vi "One Chart Temple.vi"() -> ()   [LabVIEW 2015]
doc: "该连续测量范例项目在队列消息处理器模板的基础上实现。\n\n事件处理循环负责按用户界面操作生成对应的消息。\n\n消息处理循环负责对事件处理循环或其他消息生成的消息进行处理。其中还包括用于采集和记录消息处理循环的子VI，以及用于更新图表的循环。"
uses:
  Settings/Settings.ctl
  Acquisition/Hardware Configuration.ctl
  Logging/Logging Configuration.ctl
  controls/UI Data.ctl
  controls/UI State.ctl
  support/Message Queue/Enqueue Message (Single).vi
  <vilib>/Utility/error.llb/Error Cluster From Error Code.vi
  <vilib>/ErrorRing/Error Ring.xnode
  Acquisition/Acquisition.lvlib
  Logging/Logging.lvlib
  Settings/Settings.lvlib
  support/User Event - Stop/User Event - Stop.lvlib
  support/Message Queue/Message Queue.lvlib
  Motor Control/Motor Control.lvlib
panel:
  out "XY Graph":cluster{"Y":dbl[], "Y":dbl[]}[](graph) caption="XY图"
  in  "清零":bool
  in  "读取":bool
  out "模拟通道5":dbl
  out "模拟通道4":dbl
  out "模拟通道3":dbl
  out "模拟通道2":dbl
  out "模拟通道1":dbl
  out "模拟通道0":dbl
  out "角度":dbl
  in  "计算":bool
  in  "Start":bool caption="开始"
  in  "Stop":bool caption="停止"
  out "Status":string caption="状态"
  in  "Exit":bool caption="退出"
  # "测量项目"
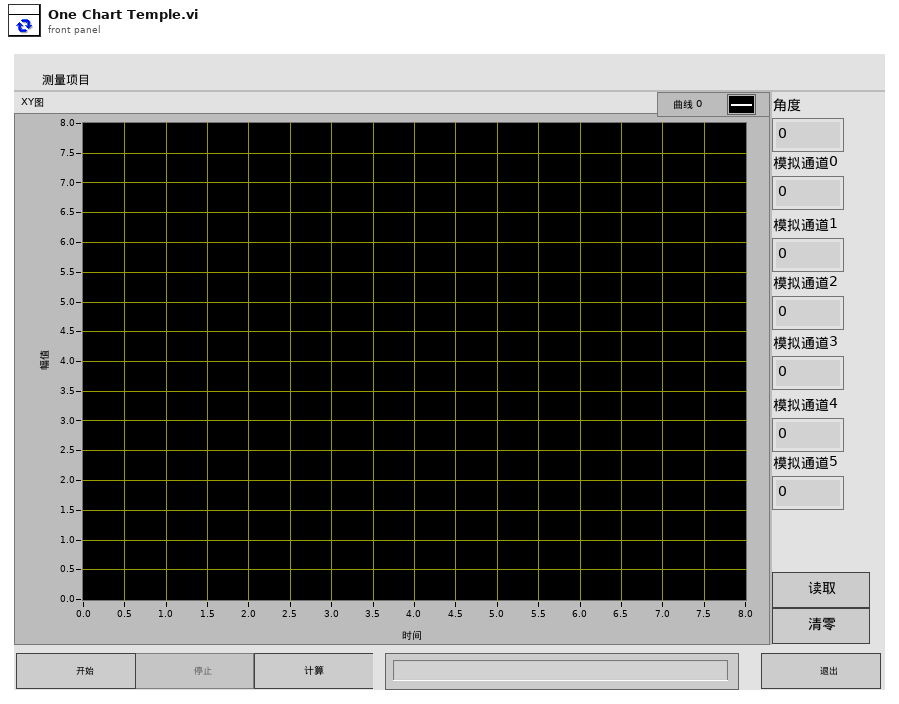
[diagram p1: front panel]
types:
  T1 = typedef "UI State.ctl" = enum16{"Idle", "Acquiring and Logging", "Waiting for Exit", "Waiting for Exit (Acq Stopped)", "Waiting for Exit (Log Stopped)", "Waiting for Stop", "Waiting for Stop (Acq Stopped)", "Waiting for Stop (Log Stopped)"}
  T2 = typedef "UI Data.ctl" = cluster{"Start Ref":refnum<vi>, "Stop Ref":refnum<vi>, "calculate Ref":refnum<vi>, "Status Ref":refnum<vi>, "Exit Ref":refnum<vi>, "Data Ref":refnum<vi>, "read Ref":refnum<vi>, "clean Ref":refnum<vi>}
  T3 = typedef "Settings.lvlib/Settings.ctl" = cluster{"Hardware Configuration":T4, "Logging Configuration":T5}
  T4 = typedef "Acquisition.lvlib/Hardware Configuration.ctl" = cluster{"电压读取设置":cluster{"DAQmx Channel":tag, "Max Input":dbl, "Min Input":dbl, "Sample Rate":dbl, "Sample Number":i32, "DAQmx Task":refnum<k21>}, "角度传感器设置":cluster{"counter":tag, "units":i32, "分辨率":i32, "初始角度":dbl, "DecodingType":i32, "A相端口":tag, "B相端口":tag, "task in":refnum<k21>}}
  T5 = typedef "Logging.lvlib/Logging Configuration.ctl" = cluster{"Log File Base Path":path, "电压传感器转换率":dbl[], "电压传感器本底":dbl[]}
  T6 = typedef "Message Queue.lvlib/All Message Queues.ctl" = cluster{"UI":refnum<queue>, "Acquisition":refnum<queue>, "Logging":refnum<queue>, "MotorCtrl":refnum<queue>, "plot logic":refnum<queue>}
  T7 = enum8{"Enabled", "Disabled", "Disabled and Grayed Out"}
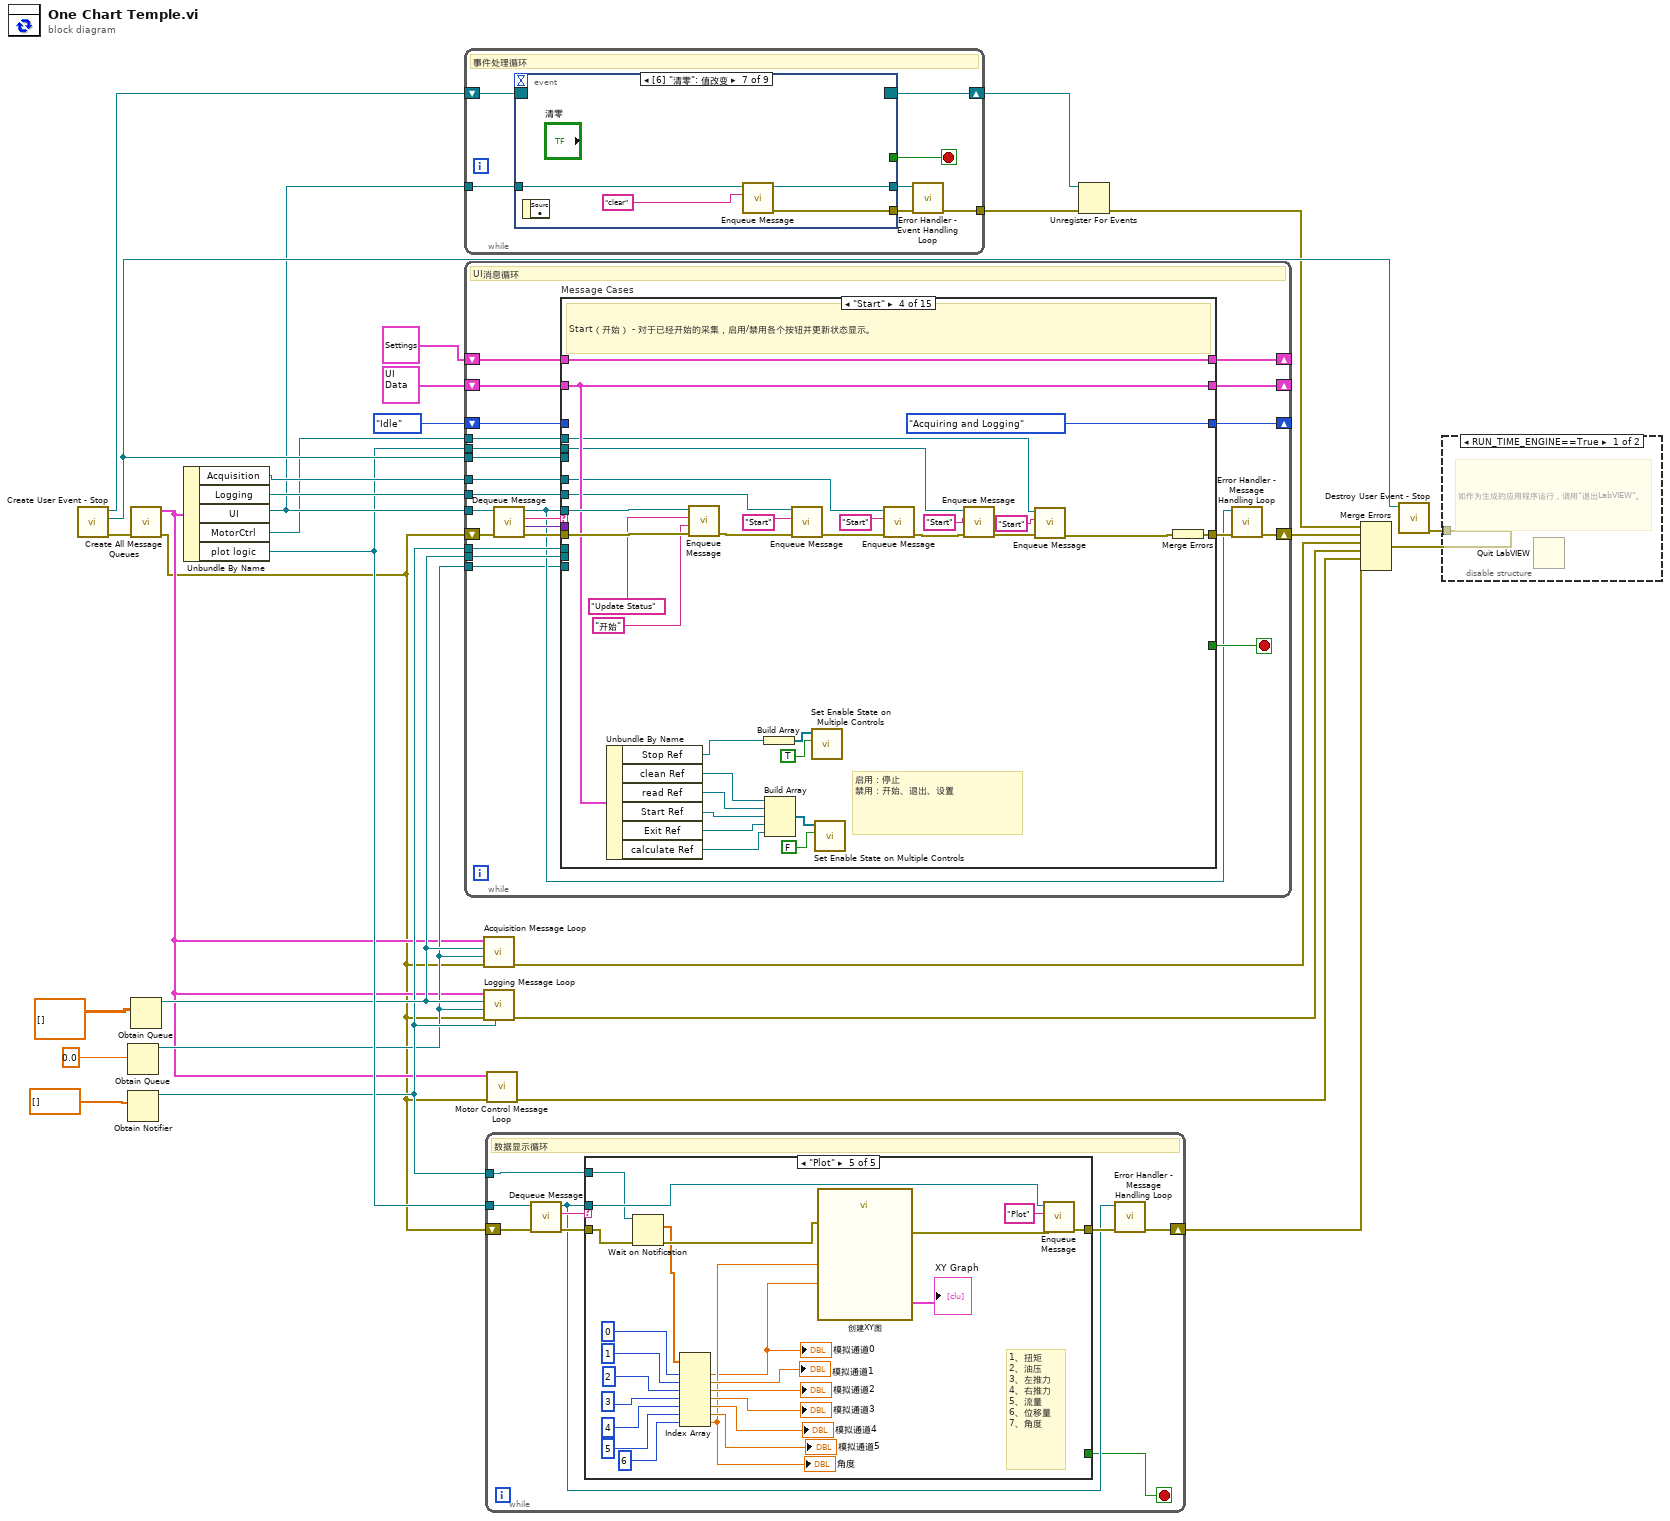
[diagram p0: block diagram]
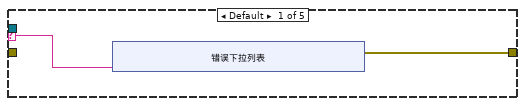
[diagram p3: hidden frame]
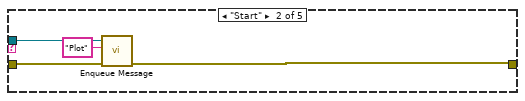
[diagram p4: hidden frame]
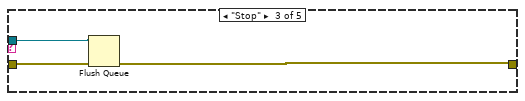
[diagram p5: hidden frame]
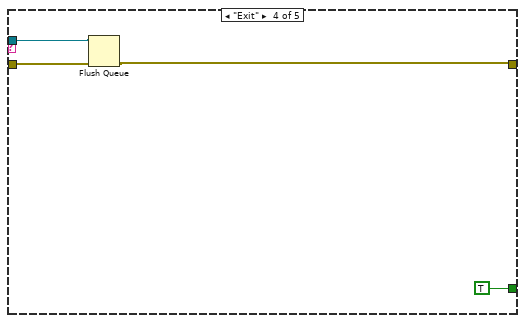
[diagram p6: hidden frame]
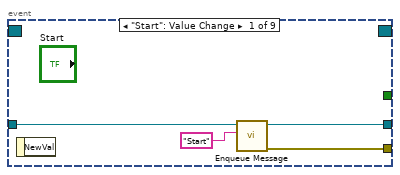
[diagram p7: hidden frame]
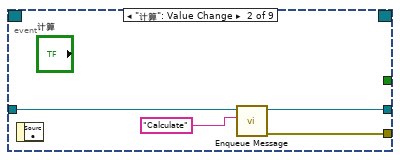
[diagram p8: hidden frame]
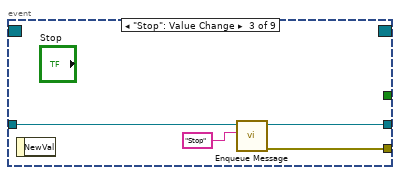
[diagram p9: hidden frame]
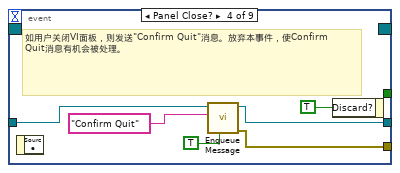
[diagram p10: hidden frame]
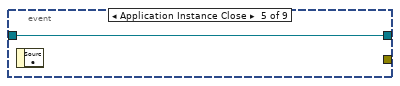
[diagram p11: hidden frame]
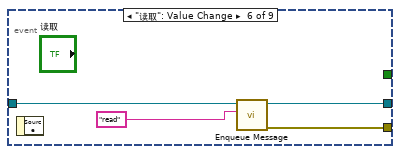
[diagram p12: hidden frame]
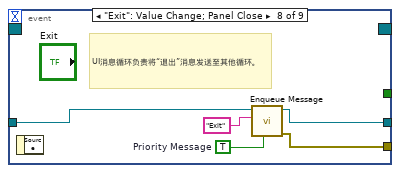
[diagram p13: hidden frame]
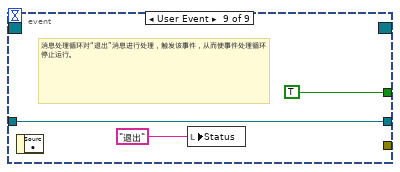
[diagram p14: hidden frame]
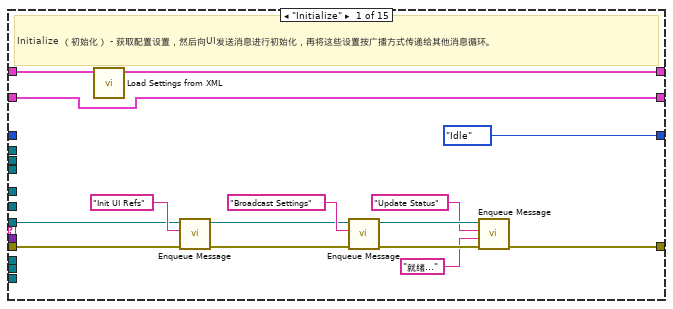
[diagram p15: hidden frame]
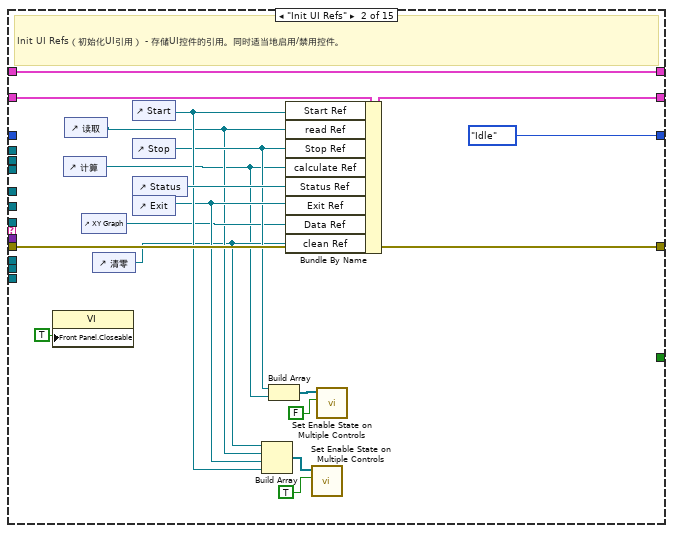
[diagram p16: hidden frame]
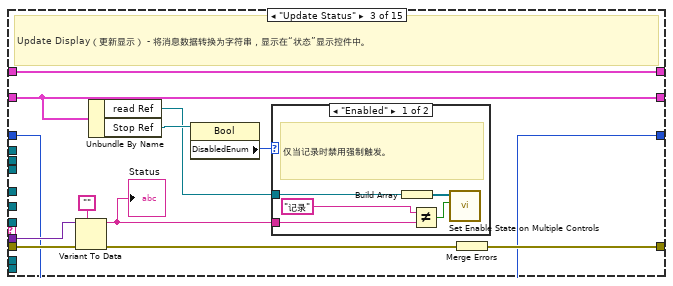
[diagram p17: hidden frame]
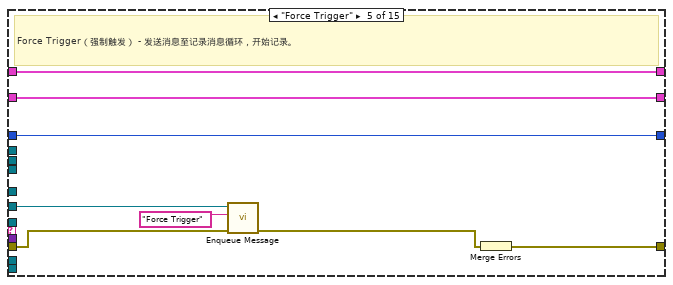
[diagram p19: hidden frame]
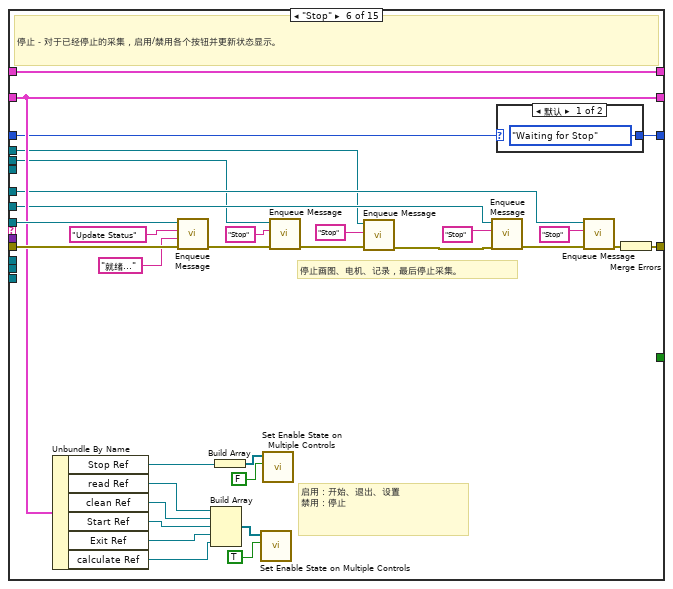
[diagram p20: hidden frame]
diagram:
  n1 = call "Create User Event - Stop.vi"() -> ("error out"=w23:errorcluster, "User Event - Stop"=w25:refnum<user-event>, "Stop Event Registration Refnum"=w26:refnum<event-registration>)  [unwired: 9 in]
  n2 = Obtain Queue(element data type=0.0) -> (queue out=w5:refnum<queue>)  [unwired: 4 in, 2 out]
  n3 = Obtain Notifier(notification data type=dbl[] []) -> (notifier out=w7:refnum<notifier>)  [unwired: 3 in, 2 out]
  n4 = call "Create All Message Queues.vi"("error in (no error)"=w23) -> ("error out"=w3:errorcluster, "Message Queues out"=w4:T6)  [unwired: 9 in]
  n5 = Obtain Queue(element data type=dbl[][] []) -> (queue out=w8:refnum<queue>)  [unwired: 4 in, 2 out]
  n6 = Unbundle By Name(w4) -> ("Acquisition"=w17:refnum<queue>, "Logging"=w16:refnum<queue>, "UI"=w15:refnum<queue>, "MotorCtrl"=w12:refnum<queue>, "plot logic"=w11:refnum<queue>)
  n7 = while {
    tunnel: w15 -> [w35]
    tunnel: [w30] -> w28
    shift-right: [w34] -> w19
    shift-left: w26 -> [w36]
    stop <- w33 stop-if-true
    # "事件处理循环"
    n8 = event shown="[6] \"清零\": 值改变" {
      selector: w36 -> [_ _ _ _ _ _ _ _ _]
      dyn-events: [_ _ _ _ _ _ _ _ _] -> w34
      timeout: _ -> [_ _ _ _ _ _ _ _ _]
      tunnel: [_ _ _ _ _ _ _ _ TRUE ("Discard?")] -> w33
      tunnel: w35 -> [w38 w43 w47 w54 w55 w57 w61 w65 w69]
      tunnel: [w40 w42 w46 w49 _ w59 w63 w68 _] -> w31
      tunnel: [w37 w41 w45 w50 w55 w56 w60 w64 w69] -> w32
      event "Start": Value Change {
        n9 = event-data() -> ()  [unwired: 1 in, 1 out]
        n10 = call-poly "Enqueue Message.vi"("Message"="Start", "Message Queue"=w38) -> ("error out"=w40:errorcluster, "dup Message Queue"=w37:refnum<queue>)  [unwired: 8 in]
      }
      event "计算": Value Change {
        n11 = event-data() -> ()  [unwired: 1 in, 1 out]
        n12 = call-poly "Enqueue Message.vi"("Message"="Calculate", "Message Queue"=w43) -> ("error out"=w42:errorcluster, "dup Message Queue"=w41:refnum<queue>)  [unwired: 8 in]
      }
      event "Stop": Value Change {
        n13 = event-data() -> ()  [unwired: 1 in, 1 out]
        n14 = call-poly "Enqueue Message.vi"("Message"="Stop", "Message Queue"=w47) -> ("error out"=w46:errorcluster, "dup Message Queue"=w45:refnum<queue>)  [unwired: 8 in]
      }
      event Panel Close? {
        # "如用户关闭VI面板，则发送\"Confirm Quit\"消息。放弃本事件，使Confirm Quit消息有机会被处理。"
        n15 = event-data() -> ()  [unwired: 1 in, 1 out]
        n16 = call-poly "Enqueue Message.vi"("Priority Message? (F)"=TRUE, "Message"="Confirm Quit", "Message Queue"=w54) -> ("error out"=w49:errorcluster, "dup Message Queue"=w50:refnum<queue>)  [unwired: 7 in]
        n17 = event-data("Discard?"=TRUE) -> ()  [unwired: 1 in, 1 out]
      }
      event Application Instance Close {
        n18 = event-data() -> ()  [unwired: 1 in, 1 out]
      }
      event "读取": Value Change {
        n19 = event-data() -> ()  [unwired: 1 in, 1 out]
        n20 = call-poly "Enqueue Message.vi"("Message"="read", "Message Queue"=w57) -> ("error out"=w59:errorcluster, "dup Message Queue"=w56:refnum<queue>)  [unwired: 8 in]
      }
      event "清零": Value Change {
        n21 = event-data() -> ()  [unwired: 1 in, 1 out]
        n22 = call-poly "Enqueue Message.vi"("Message"="clear", "Message Queue"=w61) -> ("error out"=w63:errorcluster, "dup Message Queue"=w60:refnum<queue>)  [unwired: 8 in]
      }
      event "Exit": Value Change; Panel Close {
        w66 = TRUE  # Priority Message
        # "UI消息循环负责将“退出”消息发送至其他循环。"
        n23 = event-data() -> ()  [unwired: 1 in, 1 out]
        n24 = call-poly "Enqueue Message.vi"("Priority Message? (F)"=w66, "Message"="Exit", "Message Queue"=w65) -> ("error out"=w68:errorcluster, "dup Message Queue"=w64:refnum<queue>)  [unwired: 7 in]
      }
      event User Event {
        # "消息处理循环对“退出”消息进行处理，触发该事件，从而使事件处理循环停止运行。"
        n25 = event-data() -> ()  [unwired: 1 in, 1 out]
        n26 = local write "Status"("退出" ("Exit String")) -> ()
      }
    }
    n27 = call "Error Handler - Event Handling Loop.vi"("error in (no error)"=w31, "Message Queue"=w32) -> ("dup error in"=w30:errorcluster)  [unwired: 8 in, 1 out]
  }
  n28 = while {
    tunnel: w15 -> [w88]
    tunnel: w25 -> [w93]
    shift-right: [w78] -> w29
    shift-left: w3 -> [w92]
    shift-right: [w87] -> _
    shift-left: T3 {"Hardware Configuration"={"电压读取设置"={"DAQmx Channel"="", "Max Input"=0.0, "Min Input"=0.0, "Sample Rate"=0.0, "Sample Number"=0, "DAQmx Task"=""}, "角度传感器设置"={"counter"="Dev1/ctr0", "units"=10146, "分辨率"=0, "初始角度"=0.0, "DecodingType"=10092, "A相端口"="/Dev1/PFI8", "B相端口"="/Dev1/PFI8", "task in"=""}}, "Logging Configuration"={"Log File Base Path"=path "", "电压传感器转换率"=[], "电压传感器本底"=[]}} ("Settings") -> [w86]
    shift-right: [w84] -> _
    shift-left: T2 {"Start Ref"=refnum, "Stop Ref"=refnum, "calculate Ref"=refnum, "Status Ref"=refnum, "Exit Ref"=refnum, "Data Ref"=refnum, "read Ref"=refnum, "clean Ref"=refnum} ("Measurement UI Controls") -> [w85]
    tunnel: w17 -> [w83]
    tunnel: w16 -> [w82]
    tunnel: w7 -> [w81]
    tunnel: w8 -> [w80]
    shift-right: [w75] -> _
    shift-left: UI_State."Idle" ("UI State") -> [w76]
    tunnel: w12 -> [w72]
    tunnel: w11 -> [w73]
    tunnel: w5 -> [w74]
    stop <- w94 stop-if-true
    # "UI消息循环"
    n29 = call "Dequeue Message.vi"("error in (no error)"=w92, "Message Queue"=w88) -> ("error out"=w91:errorcluster, "Message Data"=w89:variant, "Message"=w90:string, "dup Message Queue"=w77:refnum<queue>)  [unwired: 6 in]
    n30 = case "Message Cases" shown="\"Start\"" w90 {
      selector: w90 -> [_ _ _ _ _ _ _ _ _ _ _ _ _ _ w362]
      tunnel: w77 -> [w99 _ _ w174 _ w214 w218 w243 _ w285 w300 w310 w345 _ _]
      tunnel: w91 -> [w98 w127 w138 w173 w180 w213 w220 w245 w273 w287 w304 w309 w353 w360 _]
      tunnel: [w105 w127 w139 w175 w183 w215 w219 w244 w279 w282 w295 w308 w354 w359 w363] -> w79
      tunnel: [_ _ _ _ _ _ _ _ _ _ _ _ TRUE _ _] -> w94
      tunnel: w89 -> [_ _ w137 _ _ _ _ _ _ _ w303 _ _ _ _]
      tunnel: w93 -> [_ _ _ _ _ _ _ _ _ _ _ _ w352 _ _]
      tunnel: [w108 w126 w134 w172 w182 w212 w224 w249 w277 w284 w306 w313 w350 w358 w365] -> w87
      tunnel: w86 -> [w109 w126 w134 w172 w182 w212 w224 w249 w277 w288 w306 w313 w350 w358 w365]
      tunnel: w85 -> [w101 w125 w133 w169 w181 w209 w223 w248 w271 w281 w305 w312 w348 w357 w364]
      tunnel: [w101 w124 w133 w169 w181 w209 w223 w248 w271 w281 w305 w312 w348 w357 w364] -> w84
      tunnel: w83 -> [_ _ _ w157 _ w197 _ _ w270 _ _ _ w347 _ _]
      tunnel: w82 -> [_ _ _ w159 w177 w200 _ _ w269 _ _ _ w346 _ _]
      tunnel: w81 -> [_ _ _ _ _ _ _ _ _ _ _ _ w344 _ _]
      tunnel: w80 -> [_ _ _ _ _ _ _ _ _ _ _ _ w341 _ _]
      tunnel: w76 -> [_ _ w128 _ w176 w195 w222 w247 w268 w280 w294 w311 _ w356 w361]
      tunnel: [UI_State."Idle" ("UI State") UI_State."Idle" ("UI State") w128 UI_State."Acquiring and Logging" ("UI State") w176 w194 w221 w246 w268 w280 w294 w307 UI_State."Idle" ("UI State") w356 w361] -> w75
      tunnel: w74 -> [_ _ _ _ _ _ _ _ _ _ _ _ w335 _ _]
      tunnel: w73 -> [_ _ _ w151 _ w187 _ _ _ _ _ _ _ _ _]
      tunnel: w72 -> [_ _ _ w147 _ w185 _ _ _ _ _ _ _ _ _]
      frame "Initialize" {
        # "Initialize （初始化） - 获取配置设置，然后向UI发送消息进行初始化，再将这些设置按广播方式传递给其他消息循环。"
        n31 = call "Load Settings from XML.vi"("Settings in"=w109) -> ("Settings out"=w108:T3)  [unwired: 9 in, 1 out]
        n32 = call-poly "Enqueue Message.vi"("error in (no error)"=w98, "Message"="Init UI Refs", "Message Queue"=w99) -> ("error out"=w96:errorcluster, "dup Message Queue"=w97:refnum<queue>)  [unwired: 7 in]
        n33 = call-poly "Enqueue Message.vi"("error in (no error)"=w96, "Message"="Broadcast Settings", "Message Queue"=w97) -> ("error out"=w107:errorcluster, "dup Message Queue"=w106:refnum<queue>)  [unwired: 7 in]
        n34 = call-poly "Enqueue Message.vi"("error in (no error)"=w107, "Message Data"="就绪..." ("Ready..."), "Message"="Update Status", "Message Queue"=w106) -> ("error out"=w105:errorcluster)  [unwired: 6 in, 1 out]
      }
      frame "Init UI Refs" {
        # "Init UI Refs（初始化UI引用） - 存储UI控件的引用。同时适当地启用/禁用控件。"
        n35 = property class="VI"("Front Panel.Closeable"=TRUE ("Front Panel Window:Closeable")) -> ()  [unwired: 2 in, 2 out]
        n36 = control-ref of="计算"() -> (w110:refnum<vi>)
        n37 = control-ref of="读取"() -> (w112:refnum<vi>)
        n38 = control-ref of="XY Graph"() -> (w113:refnum<vi>)
        n39 = control-ref of="清零"() -> (w111:refnum<vi>)
        n40 = control-ref of="Start"() -> (w120:refnum<vi>)
        n41 = control-ref of="Stop"() -> (w116:refnum<vi>)
        n42 = control-ref of="Status"() -> (w121:refnum<vi>)
        n43 = control-ref of="Exit"() -> (w117:refnum<vi>)
        n44 = Build Array(w111, w112, w117, w120) -> (w119:refnum<vi>[])
        n45 = Build Array(w116, w110) -> (w115:refnum<vi>[])
        n46 = Bundle By Name(cluster=w125, "Start Ref"=w120, "read Ref"=w112, "Stop Ref"=w116, "calculate Ref"=w110, "Status Ref"=w121, "Exit Ref"=w117, "Data Ref"=w113, "clean Ref"=w111) -> (w124:T2)
        n47 = call "Set Enable State on Multiple Controls.vi"("Enable?"=TRUE, "Controls"=w119) -> ()  [unwired: 10 in]
        n48 = call "Set Enable State on Multiple Controls.vi"("Enable?"=FALSE, "Controls"=w115) -> ()  [unwired: 10 in]
      }
      frame "Update Status" {
        # "Update Display（更新显示） - 将消息数据转换为字符串，显示在“状态”显示控件中。"
        n49 = Variant To Data(error in=w138, type="", Variant=w137) -> (data=w130:string, error out=w135:errorcluster)
        "Status" <- w130
        n50 = Unbundle By Name(w133) -> ("read Ref"=w129:refnum<vi>, "Stop Ref"=w132:refnum<vi>)
        n51 = property class="Bool"(reference=w132) -> ("DisabledEnum"=w131:T7)  [unwired: 1 in, 2 out]
        n52 = case shown="\"Enabled\"" w131 {
          tunnel: w130 -> [w142 _]
          tunnel: w129 -> [w143 _]
          frame "Enabled" {
            # "仅当记录时禁用强制触发。"
            n53 = Build Array(w143) -> (w144:refnum<vi>[])
            n54 = Not Equal?(x="记录" ("Logging"), y=w142) -> (x != y?=w140:bool)
            n55 = call "Set Enable State on Multiple Controls.vi"("Enable?"=w140, "Controls"=w144) -> ()  [unwired: 10 in]
          }
          frame "Disabled", Default {
          }
        }
        n56 = Merge Errors(w135) -> (w139:errorcluster)
      }
      frame "Start" {
        # "启用：停止\n禁用：开始、退出、设置"
        # "Start（开始） - 对于已经开始的采集，启用/禁用各个按钮并更新状态显示。"
        n57 = Unbundle By Name(w169) -> ("Stop Ref"=w152:refnum<vi>, "clean Ref"=w153:refnum<vi>, "read Ref"=w154:refnum<vi>, "Start Ref"=w164:refnum<vi>, "Exit Ref"=w163:refnum<vi>, "calculate Ref"=w162:refnum<vi>)
        n58 = call-poly "Enqueue Message.vi"("error in (no error)"=w173, "Message Data"="开始" ("Waiting for trigger"), "Message"="Update Status", "Message Queue"=w174) -> ("error out"=w161:errorcluster)  [unwired: 6 in, 1 out]
        n59 = Build Array(w152) -> (w166:refnum<vi>[])
        n60 = Build Array(w153, w154, w164, w163, w162) -> (w167:refnum<vi>[])
        n61 = call-poly "Enqueue Message.vi"("error in (no error)"=w161, "Message"="Start", "Message Queue"=w159) -> ("error out"=w158:errorcluster)  [unwired: 7 in, 1 out]
        n62 = call "Set Enable State on Multiple Controls.vi"("Enable?"=TRUE, "Controls"=w166) -> ()  [unwired: 10 in]
        n63 = call "Set Enable State on Multiple Controls.vi"("Enable?"=FALSE, "Controls"=w167) -> ()  [unwired: 10 in]
        n64 = call-poly "Enqueue Message.vi"("error in (no error)"=w158, "Message"="Start", "Message Queue"=w157) -> ("error out"=w149:errorcluster)  [unwired: 7 in, 1 out]
        n65 = call-poly "Enqueue Message.vi"("error in (no error)"=w149, "Message"="Start", "Message Queue"=w151) -> ("error out"=w148:errorcluster)  [unwired: 7 in, 1 out]
        n66 = call-poly "Enqueue Message.vi"("error in (no error)"=w148, "Message"="Start", "Message Queue"=w147) -> ("error out"=w145:errorcluster)  [unwired: 7 in, 1 out]
        n67 = Merge Errors(w145) -> (w175:errorcluster)
      }
      frame "Force Trigger" {
        # "Force Trigger（强制触发） - 发送消息至记录消息循环，开始记录。"
        n68 = call-poly "Enqueue Message.vi"("error in (no error)"=w180, "Message"="Force Trigger", "Message Queue"=w177) -> ("error out"=w179:errorcluster)  [unwired: 7 in, 1 out]
        n69 = Merge Errors(w179) -> (w183:errorcluster)
      }
      frame "Stop" {
        # "停止画图、电机、记录，最后停止采集。"
        # "启用：开始、退出、设置\n禁用：停止"
        # "停止－对于已经停止的采集，启用/禁用各个按钮并更新状态显示。"
        n70 = Unbundle By Name(w209) -> ("Stop Ref"=w191:refnum<vi>, "read Ref"=w192:refnum<vi>, "clean Ref"=w193:refnum<vi>, "Start Ref"=w204:refnum<vi>, "Exit Ref"=w203:refnum<vi>, "calculate Ref"=w202:refnum<vi>)
        n71 = call-poly "Enqueue Message.vi"("error in (no error)"=w213, "Message Data"="就绪..." ("Ready..."), "Message"="Update Status", "Message Queue"=w214) -> ("error out"=w190:errorcluster)  [unwired: 6 in, 1 out]
        n72 = Build Array(w192, w193, w204, w203, w202) -> (w207:refnum<vi>[])
        n73 = Build Array(w191) -> (w206:refnum<vi>[])
        n74 = call "Set Enable State on Multiple Controls.vi"("Enable?"=TRUE, "Controls"=w207) -> ()  [unwired: 10 in]
        n75 = call "Set Enable State on Multiple Controls.vi"("Enable?"=FALSE, "Controls"=w206) -> ()  [unwired: 10 in]
        n76 = call-poly "Enqueue Message.vi"("error in (no error)"=w190, "Message"="Stop", "Message Queue"=w187) -> ("error out"=w189:errorcluster)  [unwired: 7 in, 1 out]
        n77 = call-poly "Enqueue Message.vi"("error in (no error)"=w189, "Message"="Stop", "Message Queue"=w185) -> ("error out"=w188:errorcluster)  [unwired: 7 in, 1 out]
        n78 = call-poly "Enqueue Message.vi"("error in (no error)"=w188, "Message"="Stop", "Message Queue"=w200) -> ("error out"=w199:errorcluster)  [unwired: 7 in, 1 out]
        n79 = case shown="默认" w195 {
          selector: w195 -> [_ w217]
          tunnel: [UI_State."Waiting for Stop" ("UI State") w217] -> w194
          frame Default {
          }
          frame "Waiting for Exit" {
          }
        }
        n80 = call-poly "Enqueue Message.vi"("error in (no error)"=w199, "Message"="Stop", "Message Queue"=w197) -> ("error out"=w198:errorcluster)  [unwired: 7 in, 1 out]
        n81 = Merge Errors(w198) -> (w215:errorcluster)
      }
      frame "Acquisition Stopped" {
        # "此处代码用于确定采集停止时采取何种操作。"
        n82 = case shown="\"Waiting for Stop (Log Stopped)\"" w222 {
          selector: w222 -> [w226 _ _ _ _]
          tunnel: [w226 UI_State."Waiting for Exit (Acq Stopped)" ("UI State") UI_State."Waiting for Stop (Acq Stopped)" ("UI State") UI_State."Idle" ("UI State") UI_State."Idle" ("UI State")] -> w221
          tunnel: w220 -> [w225 w227 w229 w235 w241]
          tunnel: [w225 w227 w229 w234 w240] -> w219
          tunnel: w218 -> [_ _ _ w233 w239]
          frame Default {
          }
          frame "Waiting for Exit", "Waiting for Exit (Acq Stopped)" {
          }
          frame "Waiting for Stop", "Waiting for Stop (Acq Stopped)" {
          }
          frame "Waiting for Exit (Log Stopped)" {
            # "如果正在等待退出且记录已结束，“采集停止”消息表示应退出。"
            n83 = call-poly "Enqueue Message.vi"("Priority Message? (F)"=TRUE, "error in (no error)"=w235, "Message"="Exit", "Message Queue"=w233) -> ("error out"=w234:errorcluster)  [unwired: 6 in, 1 out]
          }
          frame "Waiting for Stop (Log Stopped)" {
            # "当前状态为等待停止时，如已停止记录，则收到\"Acquisition Stopped\"消息时即可停止。"
            n84 = call-poly "Enqueue Message.vi"("error in (no error)"=w241, "Message Data"="Ready..." ("Message"), "Message"="Update Status", "Message Queue"=w239) -> ("error out"=w240:errorcluster)  [unwired: 6 in, 1 out]
          }
        }
      }
      frame "Logging Stopped" {
        # "此处代码用于确定记录停止时采取何种操作。"
        n85 = case shown="\"Waiting for Stop (Acq Stopped)\"" w247 {
          selector: w247 -> [w251 _ _ _ _]
          tunnel: [w251 UI_State."Waiting for Exit (Log Stopped)" ("UI State") UI_State."Waiting for Stop (Log Stopped)" ("UI State") UI_State."Idle" ("UI State") UI_State."Idle" ("UI State")] -> w246
          tunnel: w245 -> [w250 w252 w254 w260 w266]
          tunnel: [w250 w252 w254 w259 w265] -> w244
          tunnel: w243 -> [_ _ _ w258 w264]
          frame Default {
          }
          frame "Waiting for Exit", "Waiting for Exit (Log Stopped)" {
          }
          frame "Waiting for Stop", "Waiting for Stop (Log Stopped)" {
          }
          frame "Waiting for Exit (Acq Stopped)" {
            # "如果正在等待退出且采集已结束，“记录停止”消息表示应退出。"
            n86 = call-poly "Enqueue Message.vi"("Priority Message? (F)"=TRUE, "error in (no error)"=w260, "Message"="Exit", "Message Queue"=w258) -> ("error out"=w259:errorcluster)  [unwired: 6 in, 1 out]
          }
          frame "Waiting for Stop (Acq Stopped)" {
            # "如果正在等待停止且采集已结束，“记录停止”消息表示应停止。"
            n87 = call-poly "Enqueue Message.vi"("error in (no error)"=w266, "Message Data"="Ready..." ("Message"), "Message"="Update Status", "Message Queue"=w264) -> ("error out"=w265:errorcluster)  [unwired: 6 in, 1 out]
          }
        }
      }
      frame "Broadcast settings" {
        w272 = "Update Settings" ("Message")
        # "向“记录和采集”消息队列发送“更新设置”消息。"
        n88 = Unbundle By Name(w277) -> ("Hardware Configuration"=w276:T4, "Logging Configuration"=w275:T5)
        n89 = call-poly "Enqueue Message.vi"("Message Data"=w276, "Message"=w272, "Message Queue"=w270) -> ("error out"=w278:errorcluster)  [unwired: 7 in, 1 out]
        n90 = call-poly "Enqueue Message.vi"("error in (no error)"=w278, "Message Data"=w275, "Message"=w272, "Message Queue"=w269) -> ("error out"=w274:errorcluster)  [unwired: 6 in, 1 out]
        n91 = Merge Errors(w274, w273) -> (w279:errorcluster)
      }
      frame "Launch Settings Dialog" {
        # "用户单击“设置”按钮时，启动设置对话框。"
        n92 = call "Settings Dialog.vi"("error in (no error)"=w287, "Settings in"=w288) -> ("error out"=w283:errorcluster, "Cancelled?"=w286:bool, "Settings out"=w284:T3)  [unwired: 6 in, 1 out]
        n93 = case shown="假" w286 {
          tunnel: w285 -> [w292 _]
          tunnel: w283 -> [w291 w293]
          tunnel: [w290 w293] -> w282
          frame False {
            n94 = call-poly "Enqueue Message.vi"("error in (no error)"=w291, "Message"="Broadcast Settings", "Message Queue"=w292) -> ("error out"=w290:errorcluster)  [unwired: 7 in, 1 out]
          }
          frame True {
          }
        }
      }
      frame "Error" {
        # "Error - 检查错误消息数据及其响应。该消息由应用程序各循环结束处的“错误处理”VI发送。"
        n95 = Variant To Data(error in=w304, type=errorcluster {"status"=FALSE, "code"=0, "source"=""} ("error out"), Variant=w303) -> (data=w301:errorcluster, error out=w297:errorcluster)
        n96 = call <vilib>:"Simple Error Handler.vi"("error in (no error)"=w301) -> ()  [unwired: 4 in, 5 out]
        n97 = call-poly "Enqueue Message.vi"("Priority Message? (F)"=TRUE, "Message"="Exit", "Message Queue"=w300) -> ("error out"=w296:errorcluster)  [unwired: 7 in, 1 out]
        n98 = Merge Errors(w296, w297) -> (w295:errorcluster)
      }
      frame "Confirm Quit" {
        # "Confirm Quit - 该消息用于确认用户是否需要退出应用程序。"
        n99 = case shown="\"Acquiring and Logging\"" w311 {
          tunnel: w310 -> [w318 w324]
          tunnel: w309 -> [w317 w322]
          tunnel: [w314 w321] -> w308
          tunnel: [UI_State."Idle" ("UI State") w320] -> w307
          frame Default {
            # "如收到'Confirm Quit'消息时系统处于空闲状态，则不需要弹出确认提示。"
            n100 = call-poly "Enqueue Message.vi"("Priority Message? (F)"=TRUE, "error in (no error)"=w317, "Message"="Exit", "Message Queue"=w318) -> ("error out"=w314:errorcluster)  [unwired: 6 in, 1 out]
          }
          frame "Acquiring and Logging" {
            n101 = Two Button Dialog(message="采集仍在执行中，是否确定退出？" ("Confirm Quit Message"), 1:"否" ("No"), 2:"是" ("Yes")) -> (T button?=w323:bool)
            n102 = case shown="真" w323 {
              tunnel: w324 -> [_ w334]
              tunnel: w322 -> [w328 w333]
              tunnel: [w328 w332] -> w321
              tunnel: [UI_State."Acquiring and Logging" ("UI State") UI_State."Waiting for Exit" ("UI State")] -> w320
              frame False {
                # "用户不希望退出。"
              }
              frame True {
                n103 = call-poly "Enqueue Message.vi"("error in (no error)"=w333, "Message"="Stop", "Message Queue"=w334) -> ("error out"=w332:errorcluster)  [unwired: 7 in, 1 out]
              }
            }
          }
        }
      }
      frame "Exit" {
        w349 = "Exit" ("Message")
        # "不必检查错误输出。采集和记录队列可能已被释放。"
        # "停止VI。"
        # "Exit（退出）－触发用户事件，使“事件处理”循环停止运行。同时向“采集和记录”循环发送“退出”消息。"
        n104 = Release Queue(queue=w345, error in (no error)=w353) -> (error out=w343:errorcluster)  [unwired: 1 in, 2 out]
        n105 = call "Fire User Event - Stop.vi"("User Event - Stop"=w352) -> ("error out"=w351:errorcluster)  [unwired: 10 in]
        n106 = Release Notifier(notifier=w344, error in (no error)=w343) -> (error out=w342:errorcluster)  [unwired: 1 in, 2 out]
        n107 = Release Queue(queue=w341, error in (no error)=w342) -> (error out=w337:errorcluster)  [unwired: 1 in, 2 out]
        n108 = call-poly "Enqueue Message.vi"("Priority Message? (F)"=TRUE, "Message"=w349, "Message Queue"=w347) -> ()  [unwired: 7 in, 2 out]
        n109 = Release Queue(queue=w335, error in (no error)=w337) -> (error out=w336:errorcluster)  [unwired: 1 in, 2 out]
        n110 = call-poly "Enqueue Message.vi"("Priority Message? (F)"=TRUE, "Message"=w349, "Message Queue"=w346) -> ()  [unwired: 7 in, 2 out]
        n111 = Merge Errors(w351, w336) -> (w354:errorcluster)
      }
      frame "---Copy This Frame---" {
        # "如需创建新消息，可创建该帧的副本。在副本中，将本注释更改为对应消息的注释。"
        n112 = Merge Errors(w360) -> (w359:errorcluster)
      }
      frame Default {
        # "如得到的消息未经任何分支定义，则运行“默认”分支。输出程序错误。"
        n113 = xnode "错误下拉列表"("参数 0"=w362) -> ("错误输出"=w363:errorcluster)
      }
    }
    n114 = call "Error Handler - Message Handling Loop.vi"("error in (no error)"=w79, "Message Queue"=w77) -> ("dup error in"=w78:errorcluster)  [unwired: 8 in, 1 out]
  }
  n115 = call "Acquisition Message Loop.vi"("error in (no error)"=w3, "Angle Data Queue"=w5, "Analog Data Queue"=w8, "Message Queues"=w4) -> ("error out"=w24:errorcluster)  [unwired: 7 in]
  n116 = call "Logging Message Loop.vi"("数据通知器"=w7, "error in (no error)"=w3, "Angle Data Queue"=w5, "Analog Data Queue"=w8, "Message Queues"=w4) -> ("error out"=w22:errorcluster)  [unwired: 6 in]
  n117 = while "Data Display Loop" {
    tunnel: w7 -> [w374]
    tunnel: w11 -> [w381]
    shift-right: [w376] -> w1
    shift-left: w3 -> [w380]
    stop <- w373 stop-if-true
    # "数据显示循环"
    n118 = call "Dequeue Message.vi"("error in (no error)"=w380, "Message Queue"=w381) -> ("error out"=w378:errorcluster, "Message"=w377:string, "dup Message Queue"=w375:refnum<queue>)  [unwired: 6 in, 1 out]
    n119 = case shown="\"Plot\"" w377 {
      selector: w377 -> [w382 _ _ _ _]
      tunnel: [w383 w391 w396 w399 w405] -> w379
      tunnel: w378 -> [_ w394 w397 w401 w421]
      tunnel: w375 -> [_ w393 w395 w400 w424]
      tunnel: w374 -> [_ _ _ _ w422]
      tunnel: [_ _ _ TRUE _] -> w373
      frame Default {
        n120 = xnode "错误下拉列表"("参数 0"=w382) -> ("错误输出"=w383:errorcluster)
      }
      frame "Start" {
        n121 = call-poly "Enqueue Message.vi"("error in (no error)"=w394, "Message"="Plot", "Message Queue"=w393) -> ("error out"=w391:errorcluster)  [unwired: 7 in, 1 out]
      }
      frame "Stop" {
        n122 = Flush Queue(queue=w395, error in (no error)=w397) -> (error out=w396:errorcluster)  [unwired: 2 out]
      }
      frame "Exit" {
        n123 = Flush Queue(queue=w400, error in (no error)=w401) -> (error out=w399:errorcluster)  [unwired: 2 out]
      }
      frame "Plot" {
        # "1、扭矩\n2、油压\n3、左推力\n4、右推力\n5、流量\n6、位移量\n7、角度"
        n124 = Wait on Notification(notifier=w422, error in (no error)=w421) -> (notification=w402:dbl[], error out=w407:errorcluster)  [unwired: 2 in, 2 out]
        n125 = Index Array(array=w402, index #1=0 ("索引"), index #2=1 ("索引"), index #3=2 ("索引"), index #4=3 ("索引"), index #5=4 ("索引"), index #6=5 ("索引"), index #7=6 ("索引")) -> (element #1=w403:dbl, element #2=→"模拟通道1":dbl, element #3=→"模拟通道2":dbl, element #4=→"模拟通道3":dbl, element #5=→"模拟通道4":dbl, element #6=→"模拟通道5":dbl, element #7=w404:dbl)
        "角度" <- w404
        "模拟通道0" <- w403
        n126 = call "创建XY图"("error in (no error)"=w407, "Y Input"=w403, "X Input"=w404) -> ("error out"=w406:errorcluster, "XY Graph"=→"XY Graph":cluster{"X":dbl[], "Y":dbl[]}[])  [unwired: 7 in]
        n127 = call-poly "Enqueue Message.vi"("error in (no error)"=w406, "Message"="Plot", "Message Queue"=w424) -> ("error out"=w405:errorcluster)  [unwired: 7 in, 1 out]
      }
    }
    n128 = call "Error Handler - Message Handling Loop.vi"("error in (no error)"=w379, "Message Queue"=w375) -> ("dup error in"=w376:errorcluster)  [unwired: 8 in, 1 out]
  }
  n129 = call "Motor Control Message Loop.vi"("error in (no error)"=w3, "Message Queues"=w4) -> ("error out"=w2:errorcluster)  [unwired: 9 in]
  n130 = Unregister For Events(event registration refnum=w19, error in=w28) -> (error out=w20:errorcluster)
  n131 = Merge Errors(w20, w29, w24, w22, w2, w1) -> (w27:errorcluster)
  n132 = call "Destroy User Event - Stop.vi"("error in (no error)"=w27, "User Event - Stop"=w25) -> ("error out"=w14:errorcluster)  [unwired: 9 in]
  n133 = disable-structure shown="RUN_TIME_ENGINE==True" {
    disable-tunnel: w14 -> [_ _]
    frame condition #0 {
      # "如作为生成的应用程序运行，调用“退出LabVIEW”。"
      n134 = Quit LabVIEW() -> ()  [unwired: 1 in]
    }
    frame condition #1 (active) {
    }
  }
